vi "L17.vi"() -> ()   [LabVIEW 2012]
panel:
  out "sum":i32
  out "sum 2":i32
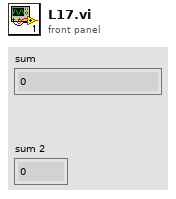
[diagram p1: front panel]
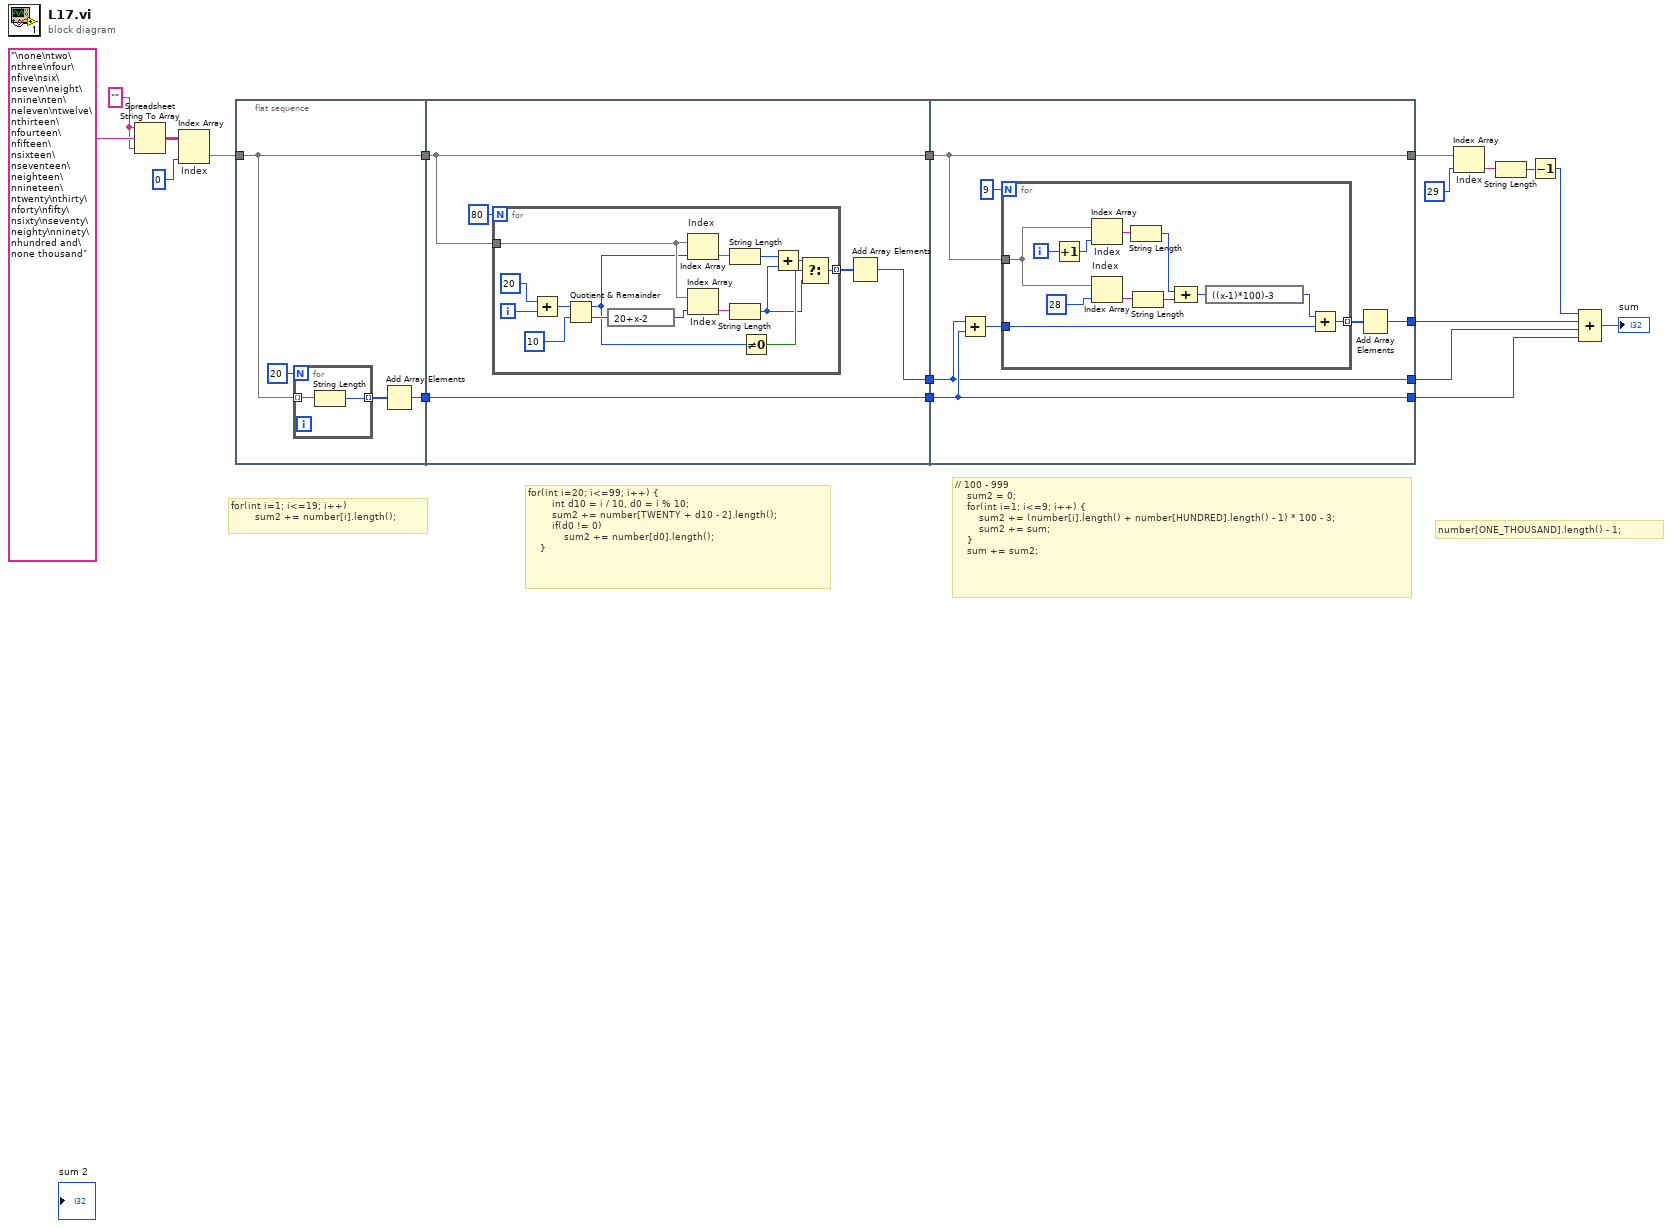
[diagram p0: block diagram]
diagram:
  w18 = "" ("spreadsheet string")
  # "for(int i=1; i<=19; i++)\n        sum2 += number[i].length();"
  # "number[ONE_THOUSAND].length() - 1;"
  # "// 100 - 999\n    sum2 = 0;\n    for(int i=1; i<=9; i++) {\n        sum2 += (number[i].length() + number[HUNDRED].length() - 1) * 100 - 3;\n        sum2 += sum;\n    }\n    sum += sum2;"
  # "for(int i=20; i<=99; i++) {\n        int d10 = i / 10, d0 = i % 10;\n        sum2 += number[TWENTY + d10 - 2].length();\n        if(d0 != 0)\n            sum2 += number[d0].length();\n    }"
  n1 = Spreadsheet String To Array(format string=w18, spreadsheet string="\none\ntwo\nthree\nfour\nfive\nsix\nseven\neight\nnine\nten\neleven\ntwelve\nthirteen\nfourteen\nfifteen\nsixteen\nseventeen\neighteen\nnineteen\ntwenty\nthirty\nforty\nfifty\nsixty\nseventy\neighty\nninety\nhundred and\none thousand", array type (2D Dbl)=w18) -> (array=w17:string[][])  [unwired: 1 in]
  n2 = Index Array "Index"(array=w17, index (col)=0 ("disabled index (col)")) -> (element=w13:string[])  [unwired: 1 in]
  n3 = flat-sequence {
    tunnel: [w21] -> w14
    tunnel: w13 -> [w21]
    tunnel: [w20] -> w10
    tunnel: w14 -> [w28]
    tunnel: [w28] -> w12
    tunnel: [w27] -> w11
    tunnel: w10 -> [w27]
    tunnel: [w26] -> w9
    tunnel: w12 -> [w46]
    tunnel: w11 -> [w48]
    tunnel: w9 -> [w47]
    tunnel: [w48] -> w1
    tunnel: [w47] -> w2
    tunnel: [w49] -> w3
    tunnel: [w46] -> w6
    frame #0 {
      n4 = for {
        N: 20 -> [_]
        tunnel: w21 -> [w24] mode=indexing
        tunnel: [w25] -> w22 mode=indexing
        n5 = String Length(string=w24) -> (length=w25:i32)
      }
      n6 = Add Array Elements(numeric array=w22) -> (sum=w20:i32)
    }
    frame #1 {
      n7 = for {
        N: 80 -> [_]
        tunnel: w28 -> [w41]
        tunnel: [w34] -> w30 mode=indexing
        i -> [w33]
        n8 = Add(x=20, y=w33) -> (x+y=w31:i32)
        n9 = Quotient & Remainder(x=w31, y=10) -> (x-y*floor(x/y)=w40:i32, floor(x/y)=w44:i32)
        n10 = expression code="20+x-2"(w44) -> (w43:i32)
        n11 = Index Array "Index"(array=w41, index=w40) -> (element=w38:string)
        n12 = Index Array "Index"(array=w41, index=w43) -> (element=w42:string)
        n13 = String Length(string=w38) -> (length=w37:i32)
        n14 = String Length(string=w42) -> (length=w36:i32)
        n15 = Not Equal To 0?(x=w40) -> (x != 0?=w39:bool)
        n16 = Add(x=w37, y=w36) -> (x+y=w35:i32)
        n17 = Select(t=w35, s=w39, f=w36) -> (s? t:f=w34:i32)
      }
      n18 = Add Array Elements(numeric array=w30) -> (sum=w26:i32)
    }
    frame #2 {
      n19 = Add(x=w47, y=w48) -> (x+y=w52:i32)
      n20 = for {
        N: 9 -> [_]
        tunnel: w46 -> [w62]
        tunnel: [w54] -> w51 mode=indexing
        tunnel: w52 -> [w55]
        i -> [w64]
        n21 = Increment(x=w64) -> (x+1=w63:i32)
        n22 = Index Array "Index"(array=w62, index=w63) -> (element=w57:string)
        n23 = Index Array "Index"(array=w62, index=28) -> (element=w60:string)
        n24 = String Length(string=w57) -> (length=w59:i32)
        n25 = String Length(string=w60) -> (length=w58:i32)
        n26 = Compound Arithmetic op=ADD(w59, w58) -> (w53:i32)
        n27 = expression code="((x-1)*100)-3"(w53) -> (w56:i32)
        n28 = Add(x=w56, y=w55) -> (x+y=w54:i32)
      }
      n29 = Add Array Elements(numeric array=w51) -> (sum=w49:i32)
    }
  }
  n30 = Index Array "Index"(array=w6, index=29) -> (element=w5:string)
  n31 = String Length(string=w5) -> (length=w7:i32)
  n32 = Decrement(x=w7) -> (x-1=w4:i32)
  n33 = Compound Arithmetic op=ADD(w4, w3, w2, w1) -> (→"sum":i32)
